vi "_TangoExceptionToLabviewError.vi"(1 "error in":errorcluster, 2 "location":string="[unknown location]", 3 "error stack":string[](array[string])=["noError", "noError", "noError"], 4 "error code":i32) -> (0 "error out":errorcluster)   [LabVIEW 2014, in "tango.lvlib"]
uses:
  tango.lvlib
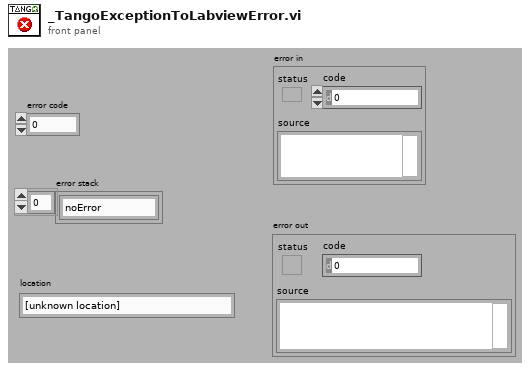
[diagram p1: front panel]
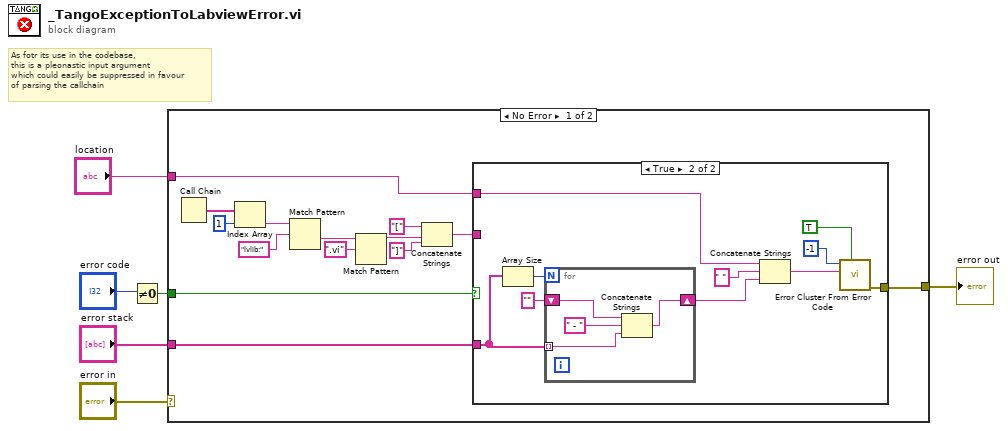
[diagram p0: block diagram]
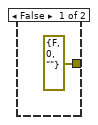
[diagram p2: hidden frame]
diagram:
  # "As fotr its use in the codebase,\nthis is a pleonastic input argument\nwhich could easily be suppressed in favour\nof parsing the callchain"
  n1 = Not Equal To 0?(x="error code") -> (x != 0?=w3:bool)
  n2 = case shown="No Error" "error in" {
    selector: "error in" -> [_ w36]
    tunnel: [w20 w36] -> w6
    tunnel: w3 -> [w19 _]
    tunnel: "error stack" -> [w18 _]
    tunnel: "location" -> [w7 _]
    frame No Error {
      n3 = Call Chain() -> (call chain=w9:string[])
      n4 = Index Array(array=w9, index=1) -> (element=w11:string)
      n5 = Match Pattern(string=w11, regular expression="lvlib:") -> (after substring=w13:string)  [unwired: 1 in, 3 out]
      n6 = Match Pattern(string=w13, regular expression=".vi") -> (before substring=w15:string)  [unwired: 1 in, 3 out]
      n7 = Concatenate Strings("[" ("string"), w15, "]" ("string")) -> (w8:string)
      n8 = case shown="True" w19 {
        tunnel: w18 -> [_ w28]
        tunnel: w7 -> [_ w27]
        tunnel: [errorcluster {"status"=FALSE, "code"=0, "source"=""} ("error in 2") w24] -> w20
        tunnel: w8 -> [_ _]
        frame False {
        }
        frame True {
          n9 = Array Size(array=w28) -> (size(s)=w31:i32)
          n10 = for {
            N: w31 -> [_]
            tunnel: w28 -> [w34] mode=indexing
            shift-right: [w32] -> w29
            shift-left: "" -> [w35]
            n11 = Concatenate Strings(w35, " - " ("string"), w34) -> (w32:string)
          }
          n12 = Concatenate Strings(w27, " " ("string"), w29) -> (w25:string)
          n13 = call <vilib>:"Error Cluster From Error Code.vi"("show call chain? (False)"=TRUE, "error message (\"\")"=w25, "error code (0)"=-1) -> ("error out"=w24:errorcluster)  [unwired: 6 in]
        }
      }
    }
    frame Error {
    }
  }
  "error out" <- w6
